vi "oa_TV Init N Channels 1 Setting.vi"(0 "threshold (auto)":dbl=inf format="%.2f", 1 "missing pulses? (no:F)":bool, 2 "channel number":i32, 5 "pulse/revolution (1)":i32=1, 7 "hysteresis (0)":dbl, 9 "pulse width (2)":i32=2, 11 "slope (Rising)":u16(ring) items=["Rising", "Falling"], 12 "output interval [s]":dbl=0.001 min=0.0) -> (3 "missing pulses? out":bool[](array[boolean]), 4 "threshold out":dbl[](array[numeric]) format="%.2f", 6 "pulse/revolution out":i32[](array[numeric]), 8 "hysteresis":dbl[](array[numeric]), 10 "pulse width out":i32[](array[numeric]), 14 "output interval":dbl[](array[numeric]), 15 "slope out":u16[](array[ring]) items=["Rising", "Falling"])   [LabVIEW 2017, in "SoundVib_Torsional.lvlib"]
uses:
  <vilib>/addons/Sound and Vibration/Order Analysis/Torsional Vibration/SoundVib_Torsional.lvlib
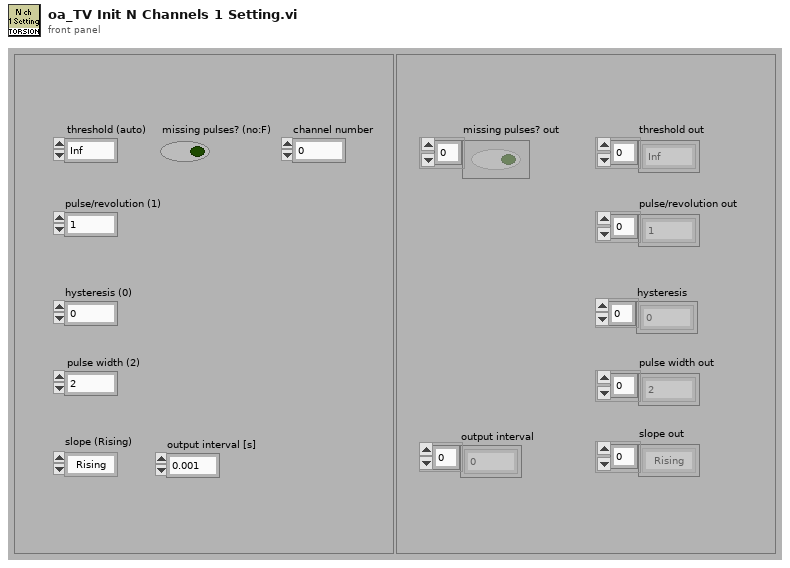
[diagram p1: front panel]
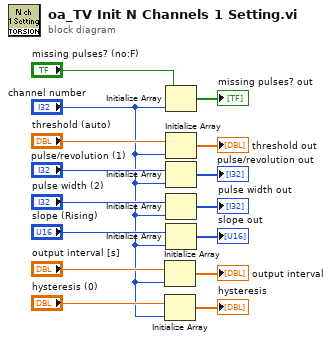
[diagram p0: block diagram]
diagram:
  n1 = Initialize Array("output interval [s]", "channel number") -> (→"output interval":dbl[])
  n2 = Initialize Array("hysteresis (0)", "channel number") -> (→"hysteresis":dbl[])
  n3 = Initialize Array("missing pulses? (no:F)", "channel number") -> (→"missing pulses? out":bool[])
  n4 = Initialize Array("threshold (auto)", "channel number") -> (→"threshold out":dbl[])
  n5 = Initialize Array("pulse/revolution (1)", "channel number") -> (→"pulse/revolution out":i32[])
  n6 = Initialize Array("pulse width (2)", "channel number") -> (→"pulse width out":i32[])
  n7 = Initialize Array("slope (Rising)", "channel number") -> (→"slope out":u16[])
